vi "Receive Control Mouse Down Event.vi"(8 "error in (no error)":errorcluster, 10 "ControlMouseDownMsg":refnum<class "ControlMouseDownMsg.lvclass">, 11 "GarphView In":refnum<class "GarphView.lvclass">) -> (0 "error out":errorcluster, 3 "GarphView Out":refnum<class "GarphView.lvclass">)   [LabVIEW 2020, in "GarphView.lvlib" / "GarphView.lvclass"]
doc: "<License>\nCopyright © 2017 Composed Systems, LLC | All rights reserved\nwww.composed.io\n\nAuthor: Ethan Stern <ethan.stern@composed.io>\n\nThis software is provided \"AS IS\" WITHOUT WARRANTIES, either express or implied, AND IS FOR EDUCATIONAL PURPOSES ONLY.\n</License>"
uses:
  GarphView.lvclass
  <vilib>/gpm_packages/@cs/mva-viewable/Source/ActorEvents/IEventAggregator Messages/ControlMouseDownMsg/ControlMouseDownMsg.lvclass
  <vilib>/gpm_packages/@cs/mva-viewable/Source/ActorEvents/IEventAggregator Messages/ControlMouseDownMsg/ControlMouseDownMsg.lvclass/ControlMouseDownMsg.ctl
  GarphView.lvclass/GarphView.ctl
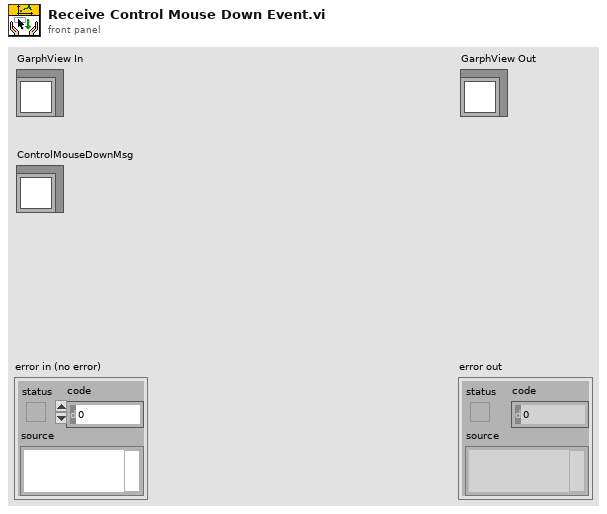
[diagram p1: front panel]
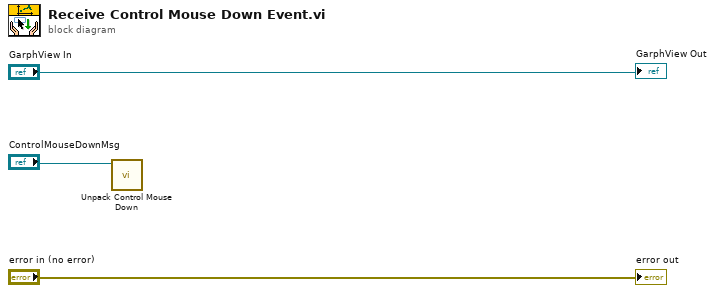
[diagram p0: block diagram]
diagram:
  n1 = call <vilib>:"Unpack Control Mouse Down.vi"("ControlMouseDownMsg"="ControlMouseDownMsg") -> ()  [unwired: 4 in, 7 out]
  "error out" <- "error in (no error)"
  "GarphView Out" <- "GarphView In"
